vi "LaserShutterTask.vi"(1 "error in (no error)":errorcluster, 2 "Laser shutter task":refnum<k21>, 3 "Command":bool) -> (0 "error out":errorcluster)   [LabVIEW 2015]
uses:
  <vilib>/DAQmx/write.llb/DAQmx Write (Digital Bool 1Line 1Point).vi
  globalVarSD.vi
  <vilib>/DAQmx/miscellaneous.llb/DAQmx Fill In Error Info.vi
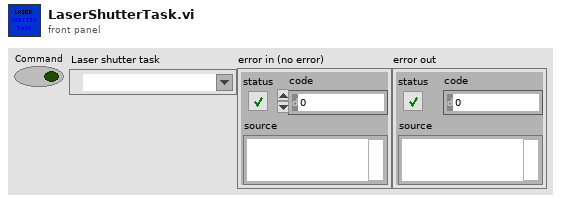
[diagram p1: front panel]
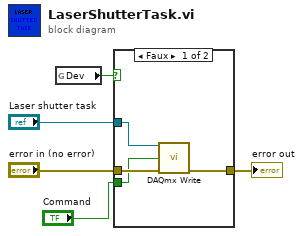
[diagram p0: block diagram]
diagram:
  n1 = global read "globalVarSD.vi" "Dev"() -> (w3:bool)
  n2 = case shown="Faux" w3 {
    tunnel: "error in (no error)" -> [w9 w10]
    tunnel: [w8 w10] -> w4
    tunnel: "Command" -> [w7 _]
    tunnel: "Laser shutter task" -> [w6 _]
    frame False {
      n3 = call-poly <vilib>:"DAQmx Write.vi"("task/channels in"=w6, "data"=w7, "error in"=w9) -> ("error out"=w8:errorcluster)  [unwired: 10 in, 2 out]
    }
    frame True {
    }
  }
  "error out" <- w4
